vi "abs.vi"(1 "Input":dbl[](array[numeric])) -> (0 "Output":dbl[](array[numeric]))   [LabVIEW 2012]
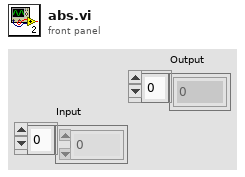
[diagram p1: front panel]
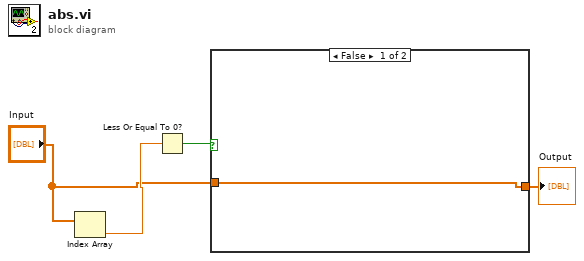
[diagram p0: block diagram]
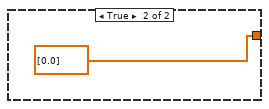
[diagram p2: hidden frame]
diagram:
  n1 = Index Array(array="Input") -> (element=w3:dbl)  [unwired: 1 in]
  n2 = Less Or Equal To 0?(x=w3) -> (x <= 0?=w2:bool)
  n3 = case shown="False" w2 {
    tunnel: [w5 dbl[] [0.0] ("subarray 3")] -> w4
    tunnel: "Input" -> [w5 _]
    frame False {
    }
    frame True {
    }
  }
  "Output" <- w4
